vi "SaveMoviePoly.vi"   [LabVIEW 2024]
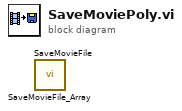
[diagram p0: block diagram]
diagram:
  n1 = call <userlib>:"SaveMovieFile_Array.vi"() -> ()  [unwired: 12 in]
  n2 = call <userlib>:"SaveMovieFile.vi"() -> ()  [unwired: 12 in]
